vi "web.vi"   [LabVIEW 2014]
uses:
  <vilib>/vision/driver/NI_Vision_Acquisition_Software.lvlib
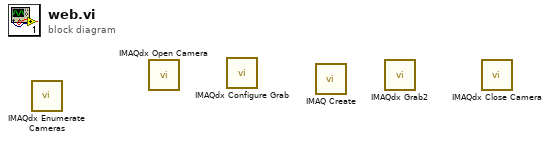
[diagram p0: block diagram]
diagram:
  n1 = call <vilib>:"IMAQdx Enumerate Cameras.vi"() -> ()  [unwired: 10 in, 2 out]
  n2 = call <vilib>:"IMAQdx Open Camera.vi"() -> ()  [unwired: 10 in, 2 out]
  n3 = call <vilib>:"IMAQdx Configure Grab.vi"() -> ()  [unwired: 10 in, 2 out]
  n4 = call "IMAQ Create"() -> ()  [unwired: 5 in, 2 out]
  n5 = call <vilib>:"IMAQdx Grab2.vi"() -> ()  [unwired: 8 in, 4 out]
  n6 = call <vilib>:"IMAQdx Close Camera.vi"() -> ()  [unwired: 11 in, 1 out]
